vi "Test Get Progress.vi"(8 "error in (no error)":errorcluster, 11 "Result Model Tests in":refnum<class "Result Model Statistics.lvclass">) -> (0 "error out":errorcluster, 3 "Result Model Tests out":refnum<class "Result Model Statistics.lvclass">)   [LabVIEW 2020, in "Result Model Statistics.lvclass"]
uses:
  Result Model Statistics.lvclass
  C:/Program Files (x86)/National Instruments/LabVIEW 2020/vi.lib/Astemes/LUnit/Test Case.lvclass
  Result/Result.ctl
  Result/Status.ctl
  Result/Type.ctl
  <vilib>/Astemes/LUnit/Test Case.lvclass/Test Case.ctl
  206db1ee-aa99-40b9-8881-171f2a77c34b.vi
  <vilib>/Astemes/LUnit/Palette/Pass.vi
  <vilib>/Astemes/LUnit/Palette/Fail.vi
  <vilib>/Astemes/LUnit/Compare Variants.vi
  <vilib>/Astemes/LUnit/Describe Comparison.vi
  <vilib>/Astemes/LUnit/Set Assertion Type.vi
  <vilib>/Astemes/LUnit/Add test result.vi
  <vilib>/Astemes/LUnit/Variant to string.vi
  <vilib>/Astemes/LUnit/LUnit Record Assertion Result.vi
  <vilib>/Astemes/LUnit/LUnit Aggregate Assertion Results.vi
  <vilib>/Astemes/LUnit/Method Result/LUnit Merge Status.vi
  <vilib>/Astemes/LUnit/LUnit Concatenate result strings.vi
  <vilib>/Utility/Data Type/Get Type Information.vi
  <vilib>/Utility/LVClass/Get LV Class Name.vi
  Result Model/Result Model.lvclass
  Result/Result.lvlib
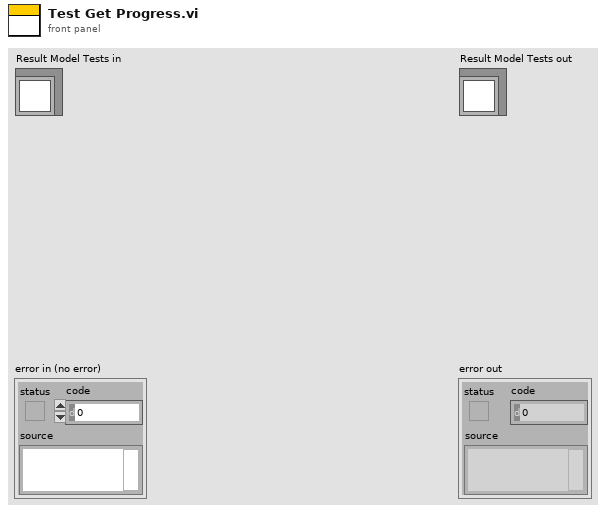
[diagram p1: front panel]
types:
  T1 = typedef "Result.lvlib/Result.ctl" = cluster{"Name":string, "Message":string, "Description":string, "Status":T2, "Result Type":T3, "Execution Time":dbl}
  T2 = typedef "Result.lvlib/Status.ctl" = enum16{"", "Passed", "Failed", "Error", "Skipped", "Setup Error", "Broken", "Teardown Error"}
  T3 = typedef "Result.lvlib/Type.ctl" = enum16{"Method", "Case", "Suite", "Pass", "Fail", "Skip", "Pass if", "Fail if", "Pass if Error", "Fail if Error", "Pass if Equal", "Fail if Equal"}
  T4 = typedef "Result Model.lvclass/Statistics.ctl" = cluster{"Method Count":u32, "Executed Methods":u32, "Passed Methods":u32, "Failed Methods":u32, "Method Errors":u32, "Skipped Method":u32, "Progress [%]":dbl}
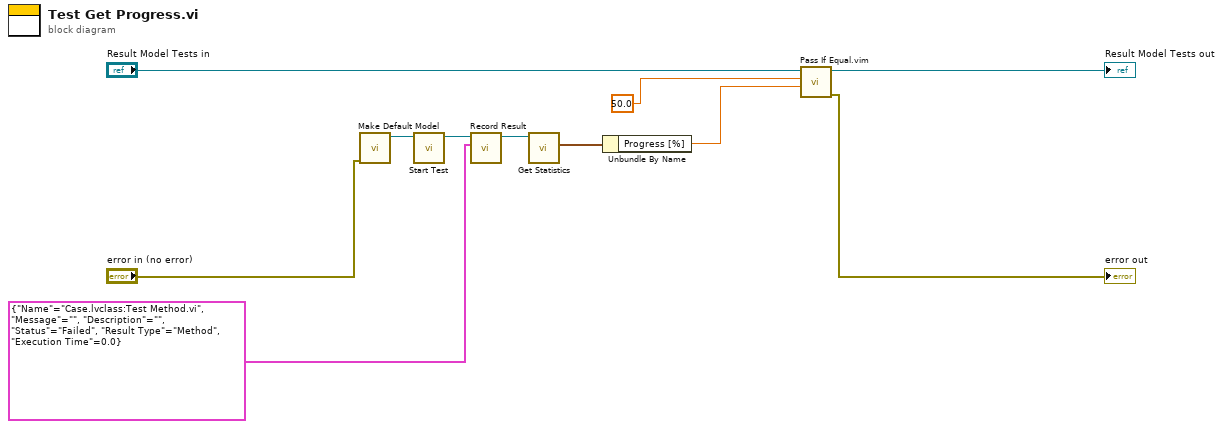
[diagram p0: block diagram]
diagram:
  n1 = call "Make Default Model.vi"("error in (no error)"="error in (no error)") -> ("Result Model out"=w10:refnum<class "Result Model.lvclass">)  [unwired: 9 in, 1 out]
  n2 = call "Start Test.vi"("Result Model In"=w10) -> ("Result Model Out"=w3:refnum<class "Result Model.lvclass">)  [unwired: 10 in]
  n3 = call "Record Result.vi"("Results"=T1 {"Name"="Case.lvclass:Test Method.vi", "Message"="", "Description"="", "Status"=enum."Failed", "Result Type"=enum."Method", "Execution Time"=0.0} ("Result"), "Result Model in"=w3) -> ("Result Model out"=w2:refnum<class "Result Model.lvclass">)  [unwired: 9 in]
  n4 = call "Get Statistics.vi"("Result Model in"=w2) -> ("Results"=w6:T4)  [unwired: 10 in]
  n5 = Unbundle By Name(w6) -> ("Progress [%]"=w5:dbl)
  n6 = call "Pass If Equal.vim"("Actual"=w5, "Expected"=50.0 ("Method Count"), "LUnit Test Case In"="Result Model Tests in") -> ("error out"=→"error out":errorcluster, "LUnit Test Case Out"=→"Result Model Tests out":refnum<class "Result Model Statistics.lvclass">)  [unwired: 7 in]
